vi "orders.vi"(8 "error in (no error)":errorcluster, 10 "Wash Options":T1, 11 "Queue in":refnum<queue>) -> (0 "error out":errorcluster, 3 "Queue out":refnum<queue>)   [LabVIEW 2015]
uses:
  USB Template (LV 8.6)/Car Wash/Controls/Wash Options.ctl
  controls/state.ctl
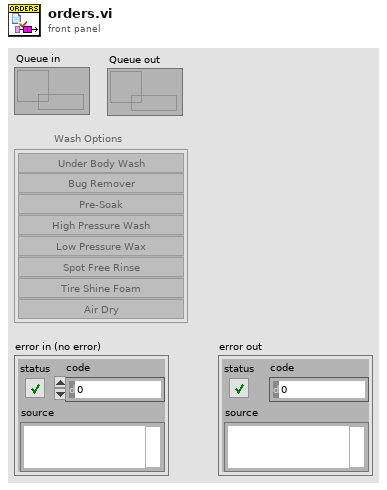
[diagram p1: front panel]
types:
  T1 = typedef "Wash Options.ctl" = cluster{"Underbody Wash":bool, "Bug Remover":bool, "Pre-Soak":bool, "High Pressure Wash":bool, "Low Pressure Wax":bool, "Spot Free Rinse":bool, "Tire Shine Foam":bool, "Air Dry":bool}
  T2 = typedef "state.ctl" = enum16{"Error", "Reset", "Exit", "Next state", "End", "Idle", "UBW", "Bug Remover", "Pre-Soak", "HPW", "LPW", "SFR", "TSF", "Air Dry", "Initialize"}
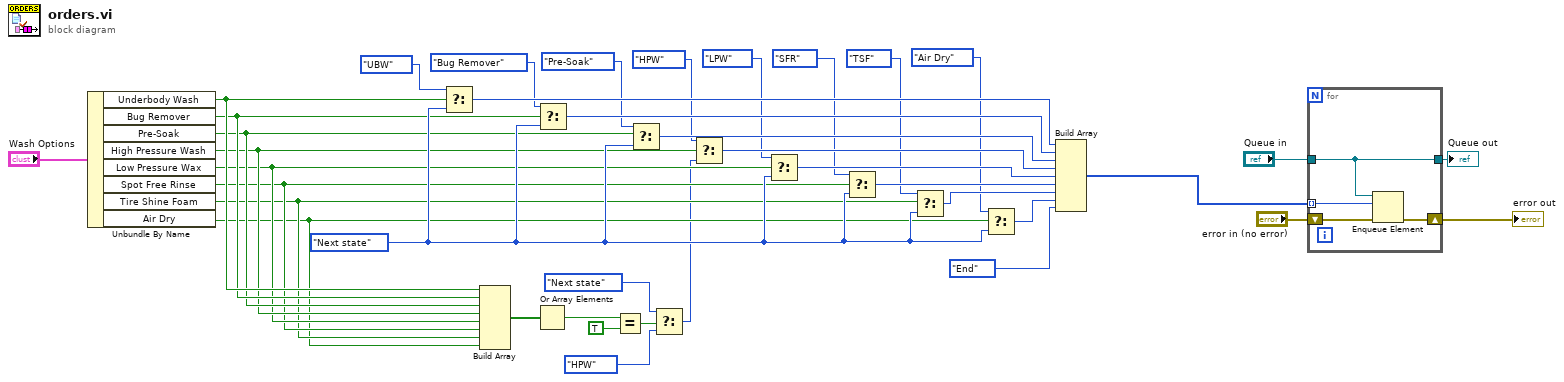
[diagram p0: block diagram]
diagram:
  w27 = state."Next state" ("state")
  n1 = Unbundle By Name("Wash Options") -> ("Underbody Wash"=w16:bool, "Bug Remover"=w15:bool, "Pre-Soak"=w14:bool, "High Pressure Wash"=w13:bool, "Low Pressure Wax"=w12:bool, "Spot Free Rinse"=w11:bool, "Tire Shine Foam"=w10:bool, "Air Dry"=w9:bool)
  n2 = Select(t=state."UBW" ("state"), s=w16, f=w27) -> (s? t:f=w31:T2)
  n3 = Build Array(w16, w15, w14, w13, w12, w11, w10, w9) -> (w8:bool[])
  n4 = Or Array Elements(Boolean array=w8) -> (logical OR=w7:bool)
  n5 = Select(t=state."Bug Remover" ("state"), s=w15, f=w27) -> (s? t:f=w32:T2)
  n6 = Equal?(x=w7, y=TRUE) -> (x = y?=w5:bool)
  n7 = Select(t=state."Pre-Soak" ("state"), s=w14, f=w27) -> (s? t:f=w33:T2)
  n8 = Select(t=state."Next state" ("state"), s=w5, f=state."HPW" ("state")) -> (s? t:f=w2:T2)
  n9 = Select(t=state."HPW" ("state"), s=w13, f=w2) -> (s? t:f=w34:T2)
  n10 = Select(t=state."LPW" ("state"), s=w12, f=w27) -> (s? t:f=w35:T2)
  n11 = Select(t=state."SFR" ("state"), s=w11, f=w27) -> (s? t:f=w36:T2)
  n12 = Select(t=state."TSF" ("state"), s=w10, f=w27) -> (s? t:f=w37:T2)
  n13 = Select(t=state."Air Dry" ("state"), s=w9, f=w27) -> (s? t:f=w38:T2)
  n14 = Build Array(w31, w32, w33, w34, w35, w36, w37, w38, state."End" ("state")) -> (w39:T2[])
  n15 = for {
    tunnel: "Queue in" -> [w40]
    shift-right: [w42] -> w30
    shift-left: "error in (no error)" -> [w43]
    tunnel: w39 -> [w41] mode=indexing
    tunnel: [w40] -> w17
    n16 = Enqueue Element(queue=w40, element=w41, error in (no error)=w43) -> (error out=w42:errorcluster)  [unwired: 1 in, 2 out]
  }
  "error out" <- w30
  "Queue out" <- w17
